vi "LuaVIEW Cleanup Handling.vi"() -> (0 "pass?":bool)   [LabVIEW 2012]
uses:
  typedefs/t_LuaVIEW Reference.ctl
panel:
  out "errors":errorcluster[](array[cluster])
  out "pass per script":bool[](array[boolean])
  out "cleanup counter":i32 caption="(synchronous)"
  in  "scripts":string[](array[string])=["-- Check cleanup on completion.\nincrement()\nlv.addcleanup(function() decrement() end)\n", "-- Check cleanup on Lua error\nincrement()\nlv.addcleanup(function() decrement() end)\nerror(\"Woof!\")", "-- Check cleanup on LabVIEW side error.\nincrement()\nlv.addcleanup(function() decrement() end)\nmsg.send(\"taskdoesnotexist\",\"garble garble\")\n", "-- Allocation function that adds its own cleanup.\nfunction allocate(amount)\n    for i=1,amount,1 do\n        increment()\n    end\n    lv.addcleanup(function()\n            for i=1,amount,1 do decrement() end\n    end)\nend\n\nallocate(666)\nallocate(42)\nerror(\"Woof!\")\nallocate(256)", "-- Allocation function that adds its own cleanup.\nfunction allocate(amount)\n    for i=1,amount,1 do\n        increment()\n    end\n    lv.addcleanup(function()\n            for i=1,amount,1 do decrement() end\n    end)\nend\n\n-- See if errors during one cleanup leaves others operational\nallocate(666)\nallocate(42)\nlv.addcleanup(function() error(\"Mooooooooooo\") end)\nallocate(256)", "-- Allocation function that adds its own cleanup.\nfunction allocate(amount)\n    for i=1,amount,1 do\n        increment()\n    end\n    lv.addcleanup(function()\n            for i=1,amount,1 do decrement() end\n    end)\nend\n\n-- See if LV errors during one cleanup leaves others operational\nallocate(666)\nallocate(42)\nlv.addcleanup(function() msg.send(\"taskdoesnotexist\", \"arf\") end)\nallocate(256)"]
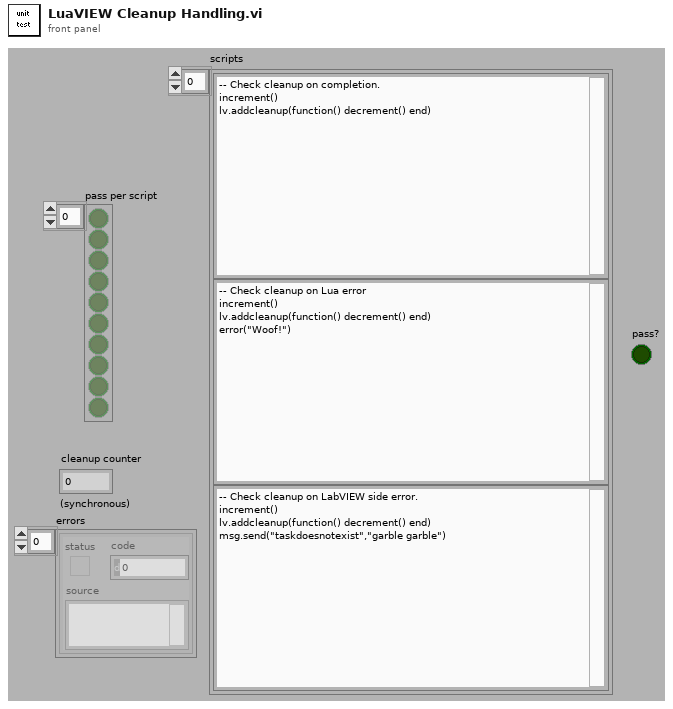
[diagram p1: front panel]
types:
  T1 = enum32{"execute", "initialize", "reset()", "increment()", "decrement()", "cleanup"}
  T2 = typedef "t_LuaVIEW Reference.ctl" = refnum<k1>
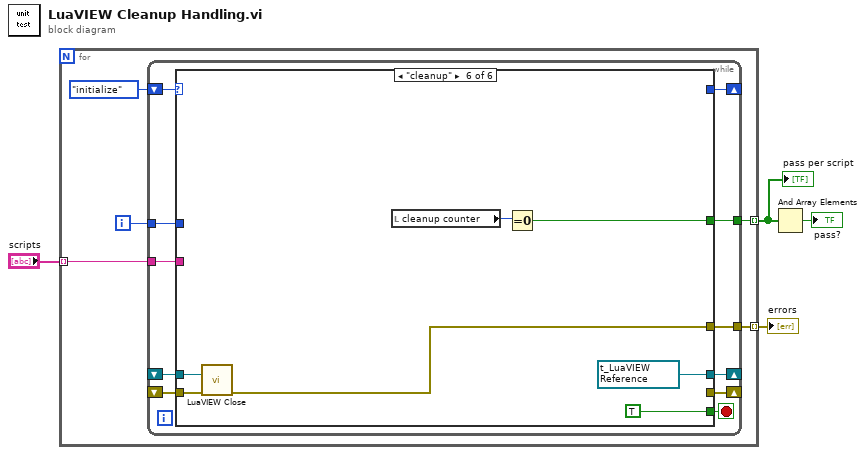
[diagram p0: block diagram]
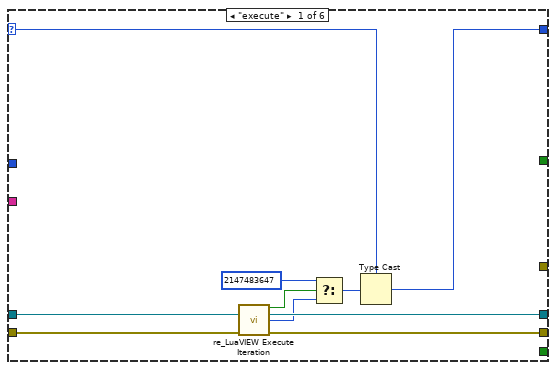
[diagram p2: hidden frame]
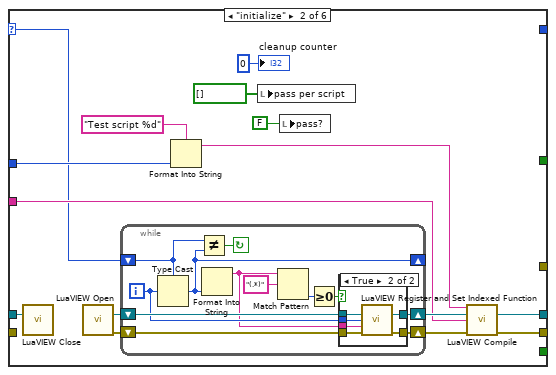
[diagram p3: hidden frame]
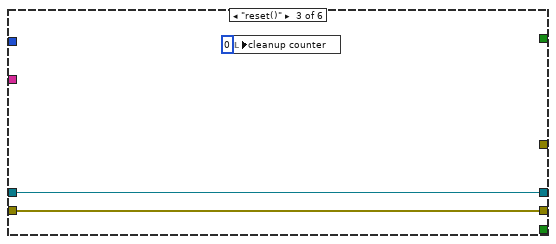
[diagram p5: hidden frame]
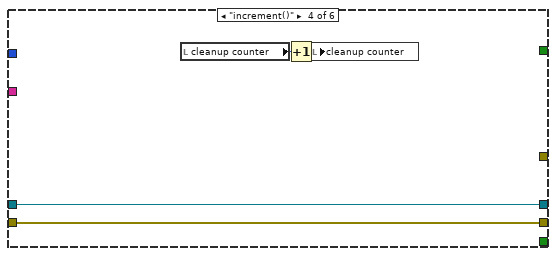
[diagram p6: hidden frame]
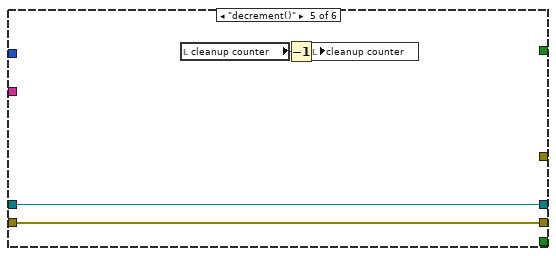
[diagram p7: hidden frame]
diagram:
  n1 = for {
    tunnel: "scripts" -> [w8] mode=indexing
    tunnel: [w7] -> w3 mode=indexing
    tunnel: [w5] -> w1 mode=indexing
    i -> [w6]
    n2 = while {
      shift-right: [w19] -> _
      shift-left: T1."initialize" -> [w12]
      shift-right: [w17] -> _
      shift-left: _ -> [w18]
      shift-right: [w16] -> _
      shift-left: _ -> [w15]
      tunnel: w8 -> [w14]
      tunnel: [w13] -> w7
      tunnel: w6 -> [w11]
      tunnel: [w10] -> w5
      stop <- w20 stop-if-true
      n3 = case shown="\"cleanup\"" w12 {
        selector: w12 -> [w23 w31 _ _ _ _]
        tunnel: [_ _ _ _ _ TRUE] -> w20
        tunnel: [w21 _ _ _ _ _] -> w19
        tunnel: w18 -> [w30 w45 w68 w72 w76 w83]
        tunnel: [w27 w40 w68 w72 w76 w82] -> w17
        tunnel: [w28 w38 w67 w71 w75 _] -> w16
        tunnel: w15 -> [w29 _ w67 w71 w75 w80]
        tunnel: w14 -> [_ w39 _ _ _ _]
        tunnel: [_ _ _ _ _ w78] -> w13
        tunnel: w11 -> [_ w36 _ _ _ _]
        tunnel: [_ _ _ _ _ w77] -> w10
        frame "execute" {
          n4 = call "re_LuaVIEW Execute Iteration.vi"("LuaVIEW reference in"=w30, "init or indexed function error"=w29) -> ("last?"=w25:bool, "LuaVIEW reference out"=w27:T2, "function index"=w26:i32, "final error"=w28:errorcluster)  [unwired: 10 in]
          n5 = Select(t=2147483647, s=w25, f=w26) -> (s? t:f=w22:i32)
          n6 = Type Cast(type=w23, x=w22) -> (*(type *) &x=w21:T1)
        }
        frame "initialize" {
          n7 = call "LuaVIEW Close.vi"("LuaVIEW reference"=w45) -> ()  [unwired: 14 in, 1 out]
          n8 = call "LuaVIEW Open.vi"() -> ("LuaVIEW reference"=w43:T2, "error out"=w44:errorcluster)  [unwired: 14 in]
          n9 = while {
            shift-right: [w51] -> w42
            shift-left: w44 -> [w54]
            shift-right: [w52] -> w41
            shift-left: w43 -> [w53]
            shift-right: [w46] -> _
            shift-left: w31 -> [w47]
            i -> [w50]
            stop <- w57 continue-if-true
            n10 = Type Cast(type=w47, x=w50) -> (*(type *) &x=w46:T1)
            n11 = Not Equal?(x=w47, y=w46) -> (x != y?=w57:bool)
            n12 = Format Into String(w46) -> (resulting string=w48:string)  [unwired: 3 in, 1 out]
            n13 = Match Pattern(string=w48, regular expression="(.*)") -> (offset past match=w55:i32)  [unwired: 1 in, 3 out]
            n14 = Greater Or Equal To 0?(x=w55) -> (x >= 0?=w49:bool)
            n15 = case shown="True" w49 {
              tunnel: w53 -> [w59 w62]
              tunnel: w50 -> [_ w63]
              tunnel: w48 -> [_ w60]
              tunnel: [w58 w65] -> w51
              tunnel: [w59 w64] -> w52
              tunnel: w54 -> [w58 w61]
              frame False {
              }
              frame True {
                n16 = call "LuaVIEW Register and Set Indexed Function.vi"("LuaVIEW reference in"=w62, "index"=w63, "synopsis"=w60, "error in (no error)"=w61) -> ("LuaVIEW reference out"=w64:T2, "error out"=w65:errorcluster)  [unwired: 10 in]
              }
            }
          }
          n17 = Format Into String(format string="Test script %d", w36) -> (resulting string=w34:string)  [unwired: 2 in, 1 out]
          n18 = local write "pass per script"(bool[] [] ("pass per script")) -> ()
          n19 = local write "pass?"(FALSE ("pass?")) -> ()
          n20 = call "LuaVIEW Compile.vi"("script name"=w34, "LuaVIEW reference in"=w41, "script"=w39, "error in (no error)"=w42) -> ("LuaVIEW reference out"=w40:T2, "error out"=w38:errorcluster)  [unwired: 10 in]
          "cleanup counter" <- 0 ("counter")
        }
        frame "reset()" {
          n21 = local write "cleanup counter"(0 ("cleanup counter")) -> ()
        }
        frame "increment()" {
          n22 = local read "cleanup counter"() -> (w70:i32)
          n23 = Increment(x=w70) -> (x+1=w69:i32)
          n24 = local write "cleanup counter"(w69) -> ()
        }
        frame "decrement()" {
          n25 = local read "cleanup counter"() -> (w74:i32)
          n26 = Decrement(x=w74) -> (x-1=w73:i32)
          n27 = local write "cleanup counter"(w73) -> ()
        }
        frame "cleanup" {
          w82 = T2 refnum items=["LuaVIEW"] ("LuaVIEW reference")
          n28 = call "LuaVIEW Close.vi"("LuaVIEW reference"=w83, "error in (no error)"=w80) -> ("dup error"=w77:errorcluster)  [unwired: 13 in]
          n29 = local read "cleanup counter"() -> (w79:i32)
          n30 = Equal To 0?(x=w79) -> (x = 0?=w78:bool)
        }
      }
    }
  }
  "pass per script" <- w3
  "errors" <- w1
  n31 = And Array Elements(Boolean array=w3) -> (logical AND=→"pass?":bool)
